vi "FPGA - PWM Example.vi"() -> ()   [LabVIEW 2013]
uses:
  <vilib>/rvi/Emulation/niFpgaSctlEmulationGetInTimedLoop.vi
  <vilib>/rvi/Emulation/niFpgaEmulationReportErrorSimple.vi
  <vilib>/rvi/Emulation/niFpgaProcessEmulError.vi
  <vilib>/rvi/Emulation/niFpgaGetClockAttributes.vi
  <vilib>/rvi/eio/common/nirviEmuTemplateMethod_errors.vi
  <vilib>/rvi/Emulation/niFpgaCriticalErrorInLSC.vi
  <vilib>/eio/EIONode/EIONode.xnode
panel:
  in  "PWM Duty Cycle (Ticks) 64":i32
  in  "PWM Duty Cycle (Ticks) 63":i32
  in  "PWM Duty Cycle (Ticks) 62":i32
  in  "PWM Duty Cycle (Ticks) 61":i32
  in  "PWM Duty Cycle (Ticks) 60":i32
  in  "PWM Duty Cycle (Ticks) 59":i32
  in  "PWM Duty Cycle (Ticks) 58":i32
  in  "PWM Duty Cycle (Ticks) 57":i32
  in  "PWM Duty Cycle (Ticks) 56":i32
  in  "PWM Duty Cycle (Ticks) 55":i32
  in  "PWM Duty Cycle (Ticks) 54":i32
  in  "PWM Duty Cycle (Ticks) 53":i32
  in  "PWM Duty Cycle (Ticks) 52":i32
  in  "PWM Duty Cycle (Ticks) 51":i32
  in  "PWM Duty Cycle (Ticks) 50":i32
  in  "PWM Duty Cycle (Ticks) 49":i32
  in  "PWM Duty Cycle (Ticks) 48":i32
  in  "PWM Duty Cycle (Ticks) 47":i32
  in  "PWM Duty Cycle (Ticks) 46":i32
  in  "PWM Duty Cycle (Ticks) 45":i32
  in  "PWM Duty Cycle (Ticks) 44":i32
  in  "PWM Duty Cycle (Ticks) 43":i32
  in  "PWM Duty Cycle (Ticks) 42":i32
  in  "PWM Duty Cycle (Ticks) 41":i32
  in  "PWM Duty Cycle (Ticks) 40":i32
  in  "PWM Duty Cycle (Ticks) 39":i32
  in  "PWM Duty Cycle (Ticks) 38":i32
  in  "PWM Duty Cycle (Ticks) 37":i32
  in  "PWM Duty Cycle (Ticks) 36":i32
  in  "PWM Duty Cycle (Ticks) 35":i32
  in  "PWM Duty Cycle (Ticks) 34":i32
  in  "PWM Duty Cycle (Ticks) 33":i32
  in  "PWM Duty Cycle (Ticks) 32":i32
  in  "PWM Duty Cycle (Ticks) 31":i32
  in  "PWM Duty Cycle (Ticks) 30":i32
  in  "PWM Duty Cycle (Ticks) 29":i32
  in  "PWM Duty Cycle (Ticks) 28":i32
  in  "PWM Duty Cycle (Ticks) 27":i32
  in  "PWM Duty Cycle (Ticks) 26":i32
  in  "PWM Duty Cycle (Ticks) 25":i32
  in  "PWM Duty Cycle (Ticks) 24":i32
  in  "PWM Duty Cycle (Ticks) 23":i32
  in  "PWM Duty Cycle (Ticks) 22":i32
  in  "PWM Duty Cycle (Ticks) 21":i32
  in  "PWM Duty Cycle (Ticks) 20":i32
  in  "PWM Duty Cycle (Ticks) 19":i32
  in  "PWM Duty Cycle (Ticks) 18":i32
  in  "PWM Duty Cycle (Ticks) 17":i32
  in  "PWM Duty Cycle (Ticks) 16":i32
  in  "PWM Duty Cycle (Ticks) 15":i32
  in  "PWM Duty Cycle (Ticks) 14":i32
  in  "PWM Duty Cycle (Ticks) 13":i32
  in  "PWM Duty Cycle (Ticks) 12":i32
  in  "PWM Duty Cycle (Ticks) 11":i32
  in  "PWM Duty Cycle (Ticks) 10":i32
  in  "PWM Duty Cycle (Ticks) 9":i32
  in  "PWM Duty Cycle (Ticks) 8":i32
  in  "PWM Duty Cycle (Ticks) 7":i32
  in  "PWM Duty Cycle (Ticks) 6":i32
  in  "PWM Duty Cycle (Ticks) 5":i32
  in  "PWM Duty Cycle (Ticks) 4":i32
  in  "PWM Duty Cycle (Ticks) 3":i32
  out "Rate (Ticks) 0..1":u32
  out "Telapsed (Ticks) 0..1":u32
  out "PWM Clock 0..1":bool
  out "9401/Slot 3 Error Code":i32
  out "stopped":bool
  in  "stop":bool
  in  "PWM Duty Cycle (Ticks) 2":i32
  in  "PWM Duty Cycle (Ticks) 1":i32
  in  "PWM Period (Ticks) 0..1":u32=40000
  # "NI 9401 PWM (Slot 3)"
  # "<- 1 Hz default"
  # "Error Codes\n65536 = Unable to communicate with module. \n65537 = Wrong module installed in slot."
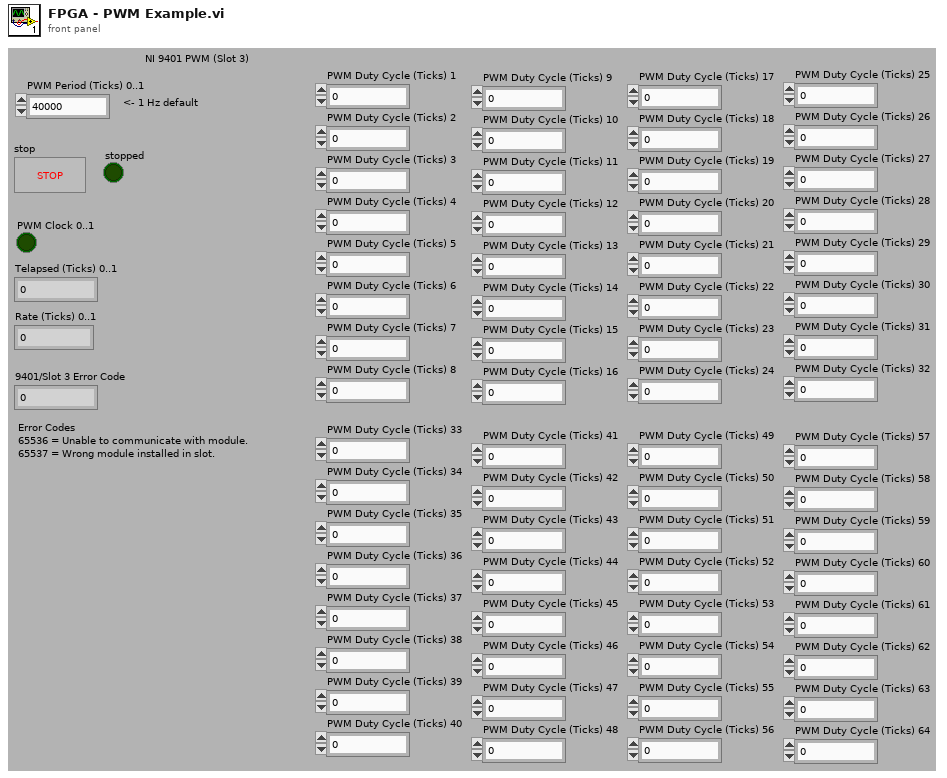
[diagram p1: front panel]
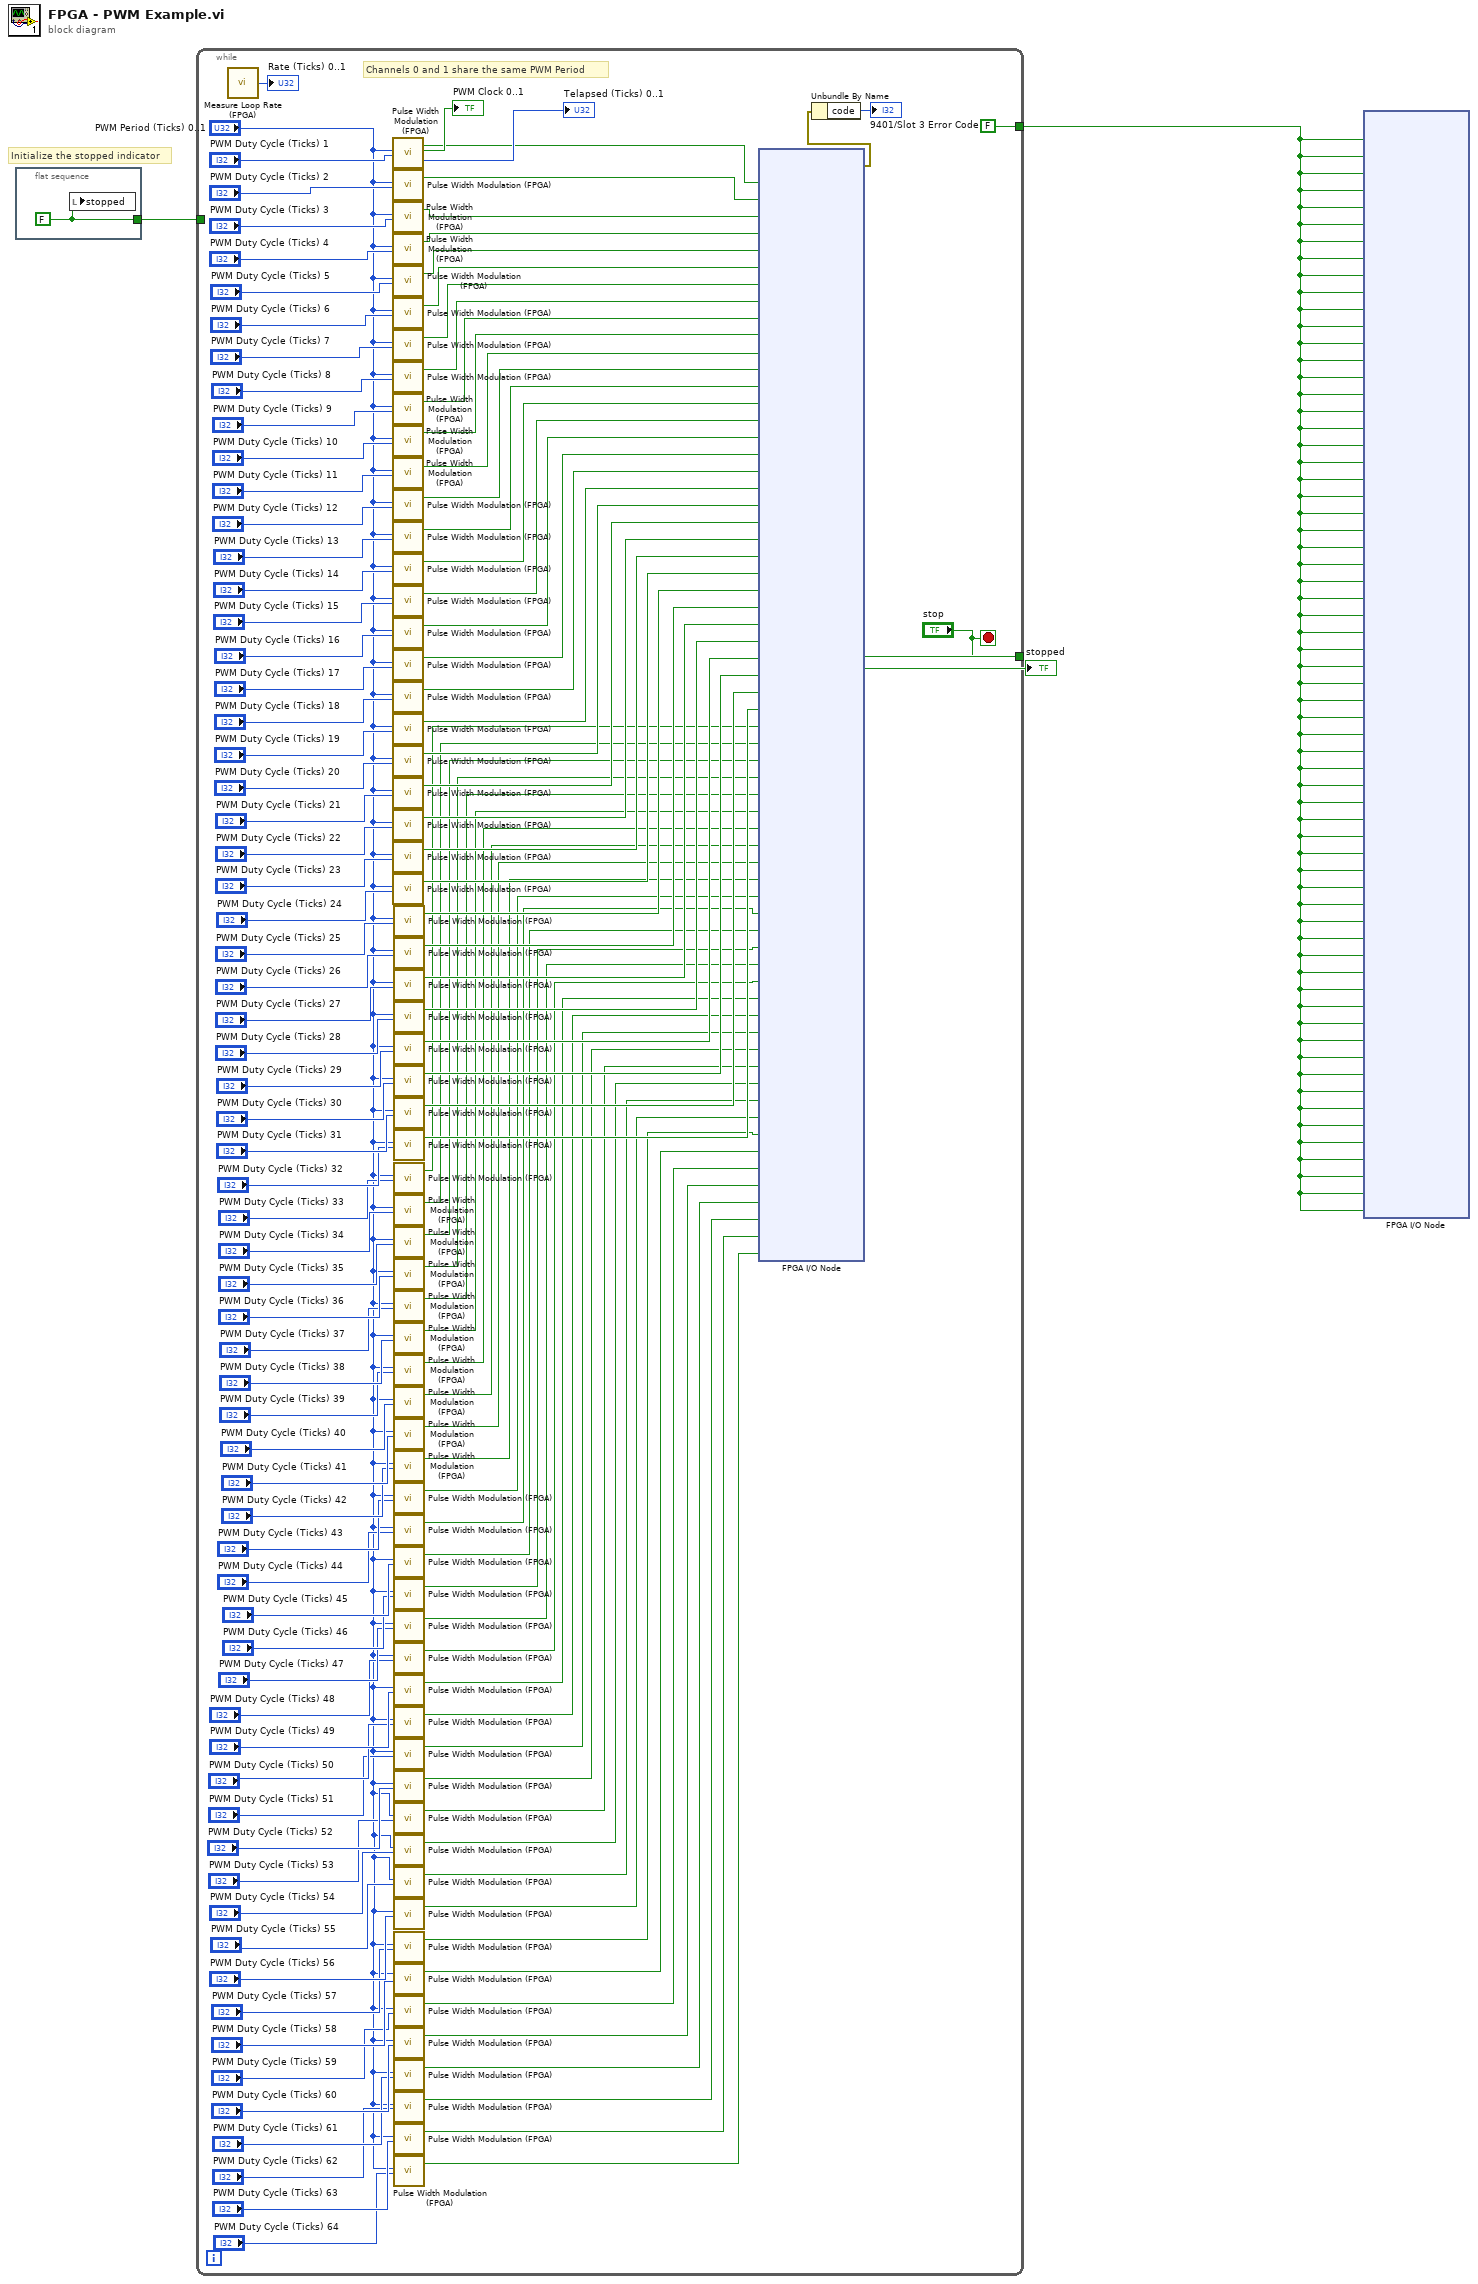
[diagram p0: block diagram]
diagram:
  # "Initialize the stopped indicator"
  n1 = flat-sequence {
    tunnel: [w4] -> w2
    frame #0 {
      w4 = FALSE ("stopped")
      n2 = local write "stopped"(w4) -> ()
    }
  }
  n3 = while {
    tunnel: [FALSE ("DO0")] -> w1
    tunnel: ["stop"] -> w3
    tunnel: w2 -> [_]
    stop <- "stop" stop-if-true
    # "Channels 0 and 1 share the same PWM Period"
    n4 = call "Measure Loop Rate (FPGA).vi"() -> ("Rate (Ticks)"=→"Rate (Ticks) 0..1":u32)  [unwired: 1 in]
    n5 = call "Pulse Width Modulation (FPGA).vi"("PWM Period (Ticks)"="PWM Period (Ticks) 0..1", "PWM Duty Cycle (Ticks)"="PWM Duty Cycle (Ticks) 1") -> ("PWM DO"=w125:bool, "PWM Clock"=→"PWM Clock 0..1":bool, "Telapsed (Ticks)"=→"Telapsed (Ticks) 0..1":u32)  [unwired: 14 in, 1 out]
    n6 = call "Pulse Width Modulation (FPGA).vi"("PWM Period (Ticks)"="PWM Period (Ticks) 0..1", "PWM Duty Cycle (Ticks)"="PWM Duty Cycle (Ticks) 2") -> ("PWM DO"=w124:bool)  [unwired: 14 in, 3 out]
    n7 = call "Pulse Width Modulation (FPGA).vi"("PWM Period (Ticks)"="PWM Period (Ticks) 0..1", "PWM Duty Cycle (Ticks)"="PWM Duty Cycle (Ticks) 3") -> ("PWM DO"=w123:bool)  [unwired: 14 in, 3 out]
    n8 = call "Pulse Width Modulation (FPGA).vi"("PWM Period (Ticks)"="PWM Period (Ticks) 0..1", "PWM Duty Cycle (Ticks)"="PWM Duty Cycle (Ticks) 4") -> ("PWM DO"=w122:bool)  [unwired: 14 in, 3 out]
    n9 = call "Pulse Width Modulation (FPGA).vi"("PWM Period (Ticks)"="PWM Period (Ticks) 0..1", "PWM Duty Cycle (Ticks)"="PWM Duty Cycle (Ticks) 5") -> ("PWM DO"=w121:bool)  [unwired: 14 in, 3 out]
    n10 = call "Pulse Width Modulation (FPGA).vi"("PWM Period (Ticks)"="PWM Period (Ticks) 0..1", "PWM Duty Cycle (Ticks)"="PWM Duty Cycle (Ticks) 6") -> ("PWM DO"=w120:bool)  [unwired: 14 in, 3 out]
    n11 = call "Pulse Width Modulation (FPGA).vi"("PWM Period (Ticks)"="PWM Period (Ticks) 0..1", "PWM Duty Cycle (Ticks)"="PWM Duty Cycle (Ticks) 7") -> ("PWM DO"=w119:bool)  [unwired: 14 in, 3 out]
    n12 = call "Pulse Width Modulation (FPGA).vi"("PWM Period (Ticks)"="PWM Period (Ticks) 0..1", "PWM Duty Cycle (Ticks)"="PWM Duty Cycle (Ticks) 8") -> ("PWM DO"=w118:bool)  [unwired: 14 in, 3 out]
    n13 = call "Pulse Width Modulation (FPGA).vi"("PWM Period (Ticks)"="PWM Period (Ticks) 0..1", "PWM Duty Cycle (Ticks)"="PWM Duty Cycle (Ticks) 9") -> ("PWM DO"=w117:bool)  [unwired: 14 in, 3 out]
    n14 = call "Pulse Width Modulation (FPGA).vi"("PWM Period (Ticks)"="PWM Period (Ticks) 0..1", "PWM Duty Cycle (Ticks)"="PWM Duty Cycle (Ticks) 10") -> ("PWM DO"=w116:bool)  [unwired: 14 in, 3 out]
    n15 = call "Pulse Width Modulation (FPGA).vi"("PWM Period (Ticks)"="PWM Period (Ticks) 0..1", "PWM Duty Cycle (Ticks)"="PWM Duty Cycle (Ticks) 11") -> ("PWM DO"=w115:bool)  [unwired: 14 in, 3 out]
    n16 = call "Pulse Width Modulation (FPGA).vi"("PWM Period (Ticks)"="PWM Period (Ticks) 0..1", "PWM Duty Cycle (Ticks)"="PWM Duty Cycle (Ticks) 12") -> ("PWM DO"=w114:bool)  [unwired: 14 in, 3 out]
    n17 = call "Pulse Width Modulation (FPGA).vi"("PWM Period (Ticks)"="PWM Period (Ticks) 0..1", "PWM Duty Cycle (Ticks)"="PWM Duty Cycle (Ticks) 13") -> ("PWM DO"=w113:bool)  [unwired: 14 in, 3 out]
    n18 = call "Pulse Width Modulation (FPGA).vi"("PWM Period (Ticks)"="PWM Period (Ticks) 0..1", "PWM Duty Cycle (Ticks)"="PWM Duty Cycle (Ticks) 14") -> ("PWM DO"=w112:bool)  [unwired: 14 in, 3 out]
    n19 = call "Pulse Width Modulation (FPGA).vi"("PWM Period (Ticks)"="PWM Period (Ticks) 0..1", "PWM Duty Cycle (Ticks)"="PWM Duty Cycle (Ticks) 15") -> ("PWM DO"=w111:bool)  [unwired: 14 in, 3 out]
    n20 = call "Pulse Width Modulation (FPGA).vi"("PWM Period (Ticks)"="PWM Period (Ticks) 0..1", "PWM Duty Cycle (Ticks)"="PWM Duty Cycle (Ticks) 16") -> ("PWM DO"=w110:bool)  [unwired: 14 in, 3 out]
    n21 = call "Pulse Width Modulation (FPGA).vi"("PWM Period (Ticks)"="PWM Period (Ticks) 0..1", "PWM Duty Cycle (Ticks)"="PWM Duty Cycle (Ticks) 17") -> ("PWM DO"=w109:bool)  [unwired: 14 in, 3 out]
    n22 = call "Pulse Width Modulation (FPGA).vi"("PWM Period (Ticks)"="PWM Period (Ticks) 0..1", "PWM Duty Cycle (Ticks)"="PWM Duty Cycle (Ticks) 18") -> ("PWM DO"=w108:bool)  [unwired: 14 in, 3 out]
    n23 = call "Pulse Width Modulation (FPGA).vi"("PWM Period (Ticks)"="PWM Period (Ticks) 0..1", "PWM Duty Cycle (Ticks)"="PWM Duty Cycle (Ticks) 19") -> ("PWM DO"=w107:bool)  [unwired: 14 in, 3 out]
    n24 = call "Pulse Width Modulation (FPGA).vi"("PWM Period (Ticks)"="PWM Period (Ticks) 0..1", "PWM Duty Cycle (Ticks)"="PWM Duty Cycle (Ticks) 20") -> ("PWM DO"=w106:bool)  [unwired: 14 in, 3 out]
    n25 = call "Pulse Width Modulation (FPGA).vi"("PWM Period (Ticks)"="PWM Period (Ticks) 0..1", "PWM Duty Cycle (Ticks)"="PWM Duty Cycle (Ticks) 21") -> ("PWM DO"=w105:bool)  [unwired: 14 in, 3 out]
    n26 = call "Pulse Width Modulation (FPGA).vi"("PWM Period (Ticks)"="PWM Period (Ticks) 0..1", "PWM Duty Cycle (Ticks)"="PWM Duty Cycle (Ticks) 22") -> ("PWM DO"=w104:bool)  [unwired: 14 in, 3 out]
    n27 = call "Pulse Width Modulation (FPGA).vi"("PWM Period (Ticks)"="PWM Period (Ticks) 0..1", "PWM Duty Cycle (Ticks)"="PWM Duty Cycle (Ticks) 23") -> ("PWM DO"=w103:bool)  [unwired: 14 in, 3 out]
    n28 = call "Pulse Width Modulation (FPGA).vi"("PWM Period (Ticks)"="PWM Period (Ticks) 0..1", "PWM Duty Cycle (Ticks)"="PWM Duty Cycle (Ticks) 24") -> ("PWM DO"=w102:bool)  [unwired: 14 in, 3 out]
    n29 = call "Pulse Width Modulation (FPGA).vi"("PWM Period (Ticks)"="PWM Period (Ticks) 0..1", "PWM Duty Cycle (Ticks)"="PWM Duty Cycle (Ticks) 25") -> ("PWM DO"=w101:bool)  [unwired: 14 in, 3 out]
    n30 = call "Pulse Width Modulation (FPGA).vi"("PWM Period (Ticks)"="PWM Period (Ticks) 0..1", "PWM Duty Cycle (Ticks)"="PWM Duty Cycle (Ticks) 26") -> ("PWM DO"=w100:bool)  [unwired: 14 in, 3 out]
    n31 = call "Pulse Width Modulation (FPGA).vi"("PWM Period (Ticks)"="PWM Period (Ticks) 0..1", "PWM Duty Cycle (Ticks)"="PWM Duty Cycle (Ticks) 27") -> ("PWM DO"=w99:bool)  [unwired: 14 in, 3 out]
    n32 = call "Pulse Width Modulation (FPGA).vi"("PWM Period (Ticks)"="PWM Period (Ticks) 0..1", "PWM Duty Cycle (Ticks)"="PWM Duty Cycle (Ticks) 28") -> ("PWM DO"=w98:bool)  [unwired: 14 in, 3 out]
    n33 = call "Pulse Width Modulation (FPGA).vi"("PWM Period (Ticks)"="PWM Period (Ticks) 0..1", "PWM Duty Cycle (Ticks)"="PWM Duty Cycle (Ticks) 29") -> ("PWM DO"=w97:bool)  [unwired: 14 in, 3 out]
    n34 = call "Pulse Width Modulation (FPGA).vi"("PWM Period (Ticks)"="PWM Period (Ticks) 0..1", "PWM Duty Cycle (Ticks)"="PWM Duty Cycle (Ticks) 30") -> ("PWM DO"=w96:bool)  [unwired: 14 in, 3 out]
    n35 = call "Pulse Width Modulation (FPGA).vi"("PWM Period (Ticks)"="PWM Period (Ticks) 0..1", "PWM Duty Cycle (Ticks)"="PWM Duty Cycle (Ticks) 31") -> ("PWM DO"=w95:bool)  [unwired: 14 in, 3 out]
    n36 = call "Pulse Width Modulation (FPGA).vi"("PWM Period (Ticks)"="PWM Period (Ticks) 0..1", "PWM Duty Cycle (Ticks)"="PWM Duty Cycle (Ticks) 32") -> ("PWM DO"=w94:bool)  [unwired: 14 in, 3 out]
    n37 = call "Pulse Width Modulation (FPGA).vi"("PWM Period (Ticks)"="PWM Period (Ticks) 0..1", "PWM Duty Cycle (Ticks)"="PWM Duty Cycle (Ticks) 33") -> ("PWM DO"=w93:bool)  [unwired: 14 in, 3 out]
    n38 = call "Pulse Width Modulation (FPGA).vi"("PWM Period (Ticks)"="PWM Period (Ticks) 0..1", "PWM Duty Cycle (Ticks)"="PWM Duty Cycle (Ticks) 34") -> ("PWM DO"=w92:bool)  [unwired: 14 in, 3 out]
    n39 = call "Pulse Width Modulation (FPGA).vi"("PWM Period (Ticks)"="PWM Period (Ticks) 0..1", "PWM Duty Cycle (Ticks)"="PWM Duty Cycle (Ticks) 35") -> ("PWM DO"=w91:bool)  [unwired: 14 in, 3 out]
    n40 = call "Pulse Width Modulation (FPGA).vi"("PWM Period (Ticks)"="PWM Period (Ticks) 0..1", "PWM Duty Cycle (Ticks)"="PWM Duty Cycle (Ticks) 36") -> ("PWM DO"=w90:bool)  [unwired: 14 in, 3 out]
    n41 = call "Pulse Width Modulation (FPGA).vi"("PWM Period (Ticks)"="PWM Period (Ticks) 0..1", "PWM Duty Cycle (Ticks)"="PWM Duty Cycle (Ticks) 37") -> ("PWM DO"=w89:bool)  [unwired: 14 in, 3 out]
    n42 = call "Pulse Width Modulation (FPGA).vi"("PWM Period (Ticks)"="PWM Period (Ticks) 0..1", "PWM Duty Cycle (Ticks)"="PWM Duty Cycle (Ticks) 38") -> ("PWM DO"=w88:bool)  [unwired: 14 in, 3 out]
    n43 = call "Pulse Width Modulation (FPGA).vi"("PWM Period (Ticks)"="PWM Period (Ticks) 0..1", "PWM Duty Cycle (Ticks)"="PWM Duty Cycle (Ticks) 39") -> ("PWM DO"=w87:bool)  [unwired: 14 in, 3 out]
    n44 = call "Pulse Width Modulation (FPGA).vi"("PWM Period (Ticks)"="PWM Period (Ticks) 0..1", "PWM Duty Cycle (Ticks)"="PWM Duty Cycle (Ticks) 40") -> ("PWM DO"=w86:bool)  [unwired: 14 in, 3 out]
    n45 = call "Pulse Width Modulation (FPGA).vi"("PWM Period (Ticks)"="PWM Period (Ticks) 0..1", "PWM Duty Cycle (Ticks)"="PWM Duty Cycle (Ticks) 41") -> ("PWM DO"=w85:bool)  [unwired: 14 in, 3 out]
    n46 = call "Pulse Width Modulation (FPGA).vi"("PWM Period (Ticks)"="PWM Period (Ticks) 0..1", "PWM Duty Cycle (Ticks)"="PWM Duty Cycle (Ticks) 42") -> ("PWM DO"=w84:bool)  [unwired: 14 in, 3 out]
    n47 = call "Pulse Width Modulation (FPGA).vi"("PWM Period (Ticks)"="PWM Period (Ticks) 0..1", "PWM Duty Cycle (Ticks)"="PWM Duty Cycle (Ticks) 43") -> ("PWM DO"=w83:bool)  [unwired: 14 in, 3 out]
    n48 = call "Pulse Width Modulation (FPGA).vi"("PWM Period (Ticks)"="PWM Period (Ticks) 0..1", "PWM Duty Cycle (Ticks)"="PWM Duty Cycle (Ticks) 44") -> ("PWM DO"=w82:bool)  [unwired: 14 in, 3 out]
    n49 = call "Pulse Width Modulation (FPGA).vi"("PWM Period (Ticks)"="PWM Period (Ticks) 0..1", "PWM Duty Cycle (Ticks)"="PWM Duty Cycle (Ticks) 45") -> ("PWM DO"=w81:bool)  [unwired: 14 in, 3 out]
    n50 = call "Pulse Width Modulation (FPGA).vi"("PWM Period (Ticks)"="PWM Period (Ticks) 0..1", "PWM Duty Cycle (Ticks)"="PWM Duty Cycle (Ticks) 46") -> ("PWM DO"=w80:bool)  [unwired: 14 in, 3 out]
    n51 = call "Pulse Width Modulation (FPGA).vi"("PWM Period (Ticks)"="PWM Period (Ticks) 0..1", "PWM Duty Cycle (Ticks)"="PWM Duty Cycle (Ticks) 47") -> ("PWM DO"=w79:bool)  [unwired: 14 in, 3 out]
    n52 = call "Pulse Width Modulation (FPGA).vi"("PWM Period (Ticks)"="PWM Period (Ticks) 0..1", "PWM Duty Cycle (Ticks)"="PWM Duty Cycle (Ticks) 48") -> ("PWM DO"=w78:bool)  [unwired: 14 in, 3 out]
    n53 = call "Pulse Width Modulation (FPGA).vi"("PWM Period (Ticks)"="PWM Period (Ticks) 0..1", "PWM Duty Cycle (Ticks)"="PWM Duty Cycle (Ticks) 49") -> ("PWM DO"=w77:bool)  [unwired: 14 in, 3 out]
    n54 = call "Pulse Width Modulation (FPGA).vi"("PWM Period (Ticks)"="PWM Period (Ticks) 0..1", "PWM Duty Cycle (Ticks)"="PWM Duty Cycle (Ticks) 50") -> ("PWM DO"=w76:bool)  [unwired: 14 in, 3 out]
    n55 = call "Pulse Width Modulation (FPGA).vi"("PWM Period (Ticks)"="PWM Period (Ticks) 0..1", "PWM Duty Cycle (Ticks)"="PWM Duty Cycle (Ticks) 51") -> ("PWM DO"=w75:bool)  [unwired: 14 in, 3 out]
    n56 = call "Pulse Width Modulation (FPGA).vi"("PWM Period (Ticks)"="PWM Period (Ticks) 0..1", "PWM Duty Cycle (Ticks)"="PWM Duty Cycle (Ticks) 52") -> ("PWM DO"=w74:bool)  [unwired: 14 in, 3 out]
    n57 = call "Pulse Width Modulation (FPGA).vi"("PWM Period (Ticks)"="PWM Period (Ticks) 0..1", "PWM Duty Cycle (Ticks)"="PWM Duty Cycle (Ticks) 53") -> ("PWM DO"=w73:bool)  [unwired: 14 in, 3 out]
    n58 = call "Pulse Width Modulation (FPGA).vi"("PWM Period (Ticks)"="PWM Period (Ticks) 0..1", "PWM Duty Cycle (Ticks)"="PWM Duty Cycle (Ticks) 54") -> ("PWM DO"=w72:bool)  [unwired: 14 in, 3 out]
    n59 = call "Pulse Width Modulation (FPGA).vi"("PWM Period (Ticks)"="PWM Period (Ticks) 0..1", "PWM Duty Cycle (Ticks)"="PWM Duty Cycle (Ticks) 55") -> ("PWM DO"=w71:bool)  [unwired: 14 in, 3 out]
    n60 = call "Pulse Width Modulation (FPGA).vi"("PWM Period (Ticks)"="PWM Period (Ticks) 0..1", "PWM Duty Cycle (Ticks)"="PWM Duty Cycle (Ticks) 56") -> ("PWM DO"=w70:bool)  [unwired: 14 in, 3 out]
    n61 = call "Pulse Width Modulation (FPGA).vi"("PWM Period (Ticks)"="PWM Period (Ticks) 0..1", "PWM Duty Cycle (Ticks)"="PWM Duty Cycle (Ticks) 57") -> ("PWM DO"=w69:bool)  [unwired: 14 in, 3 out]
    n62 = call "Pulse Width Modulation (FPGA).vi"("PWM Period (Ticks)"="PWM Period (Ticks) 0..1", "PWM Duty Cycle (Ticks)"="PWM Duty Cycle (Ticks) 58") -> ("PWM DO"=w68:bool)  [unwired: 14 in, 3 out]
    n63 = call "Pulse Width Modulation (FPGA).vi"("PWM Period (Ticks)"="PWM Period (Ticks) 0..1", "PWM Duty Cycle (Ticks)"="PWM Duty Cycle (Ticks) 59") -> ("PWM DO"=w67:bool)  [unwired: 14 in, 3 out]
    n64 = call "Pulse Width Modulation (FPGA).vi"("PWM Period (Ticks)"="PWM Period (Ticks) 0..1", "PWM Duty Cycle (Ticks)"="PWM Duty Cycle (Ticks) 60") -> ("PWM DO"=w66:bool)  [unwired: 14 in, 3 out]
    n65 = call "Pulse Width Modulation (FPGA).vi"("PWM Period (Ticks)"="PWM Period (Ticks) 0..1", "PWM Duty Cycle (Ticks)"="PWM Duty Cycle (Ticks) 61") -> ("PWM DO"=w65:bool)  [unwired: 14 in, 3 out]
    n66 = call "Pulse Width Modulation (FPGA).vi"("PWM Period (Ticks)"="PWM Period (Ticks) 0..1", "PWM Duty Cycle (Ticks)"="PWM Duty Cycle (Ticks) 62") -> ("PWM DO"=w64:bool)  [unwired: 14 in, 3 out]
    n67 = call "Pulse Width Modulation (FPGA).vi"("PWM Period (Ticks)"="PWM Period (Ticks) 0..1", "PWM Duty Cycle (Ticks)"="PWM Duty Cycle (Ticks) 63") -> ("PWM DO"=w63:bool)  [unwired: 14 in, 3 out]
    n68 = call "Pulse Width Modulation (FPGA).vi"("PWM Period (Ticks)"="PWM Period (Ticks) 0..1", "PWM Duty Cycle (Ticks)"="PWM Duty Cycle (Ticks) 64") -> ("PWM DO"=w62:bool)  [unwired: 14 in, 3 out]
    n69 = xnode "FPGA I/O Node"("Mod1/DIO0"=w125, "Mod1/DIO1"=w124, "Mod1/DIO2"=w123, "Mod1/DIO3"=w122, "Mod1/DIO4"=w121, "Mod1/DIO5"=w120, "Mod1/DIO6"=w119, "Mod1/DIO7"=w118, "Mod2/DIO0"=w117, "Mod2/DIO1"=w116, "Mod2/DIO2"=w115, "Mod2/DIO3"=w114, "Mod2/DIO4"=w113, "Mod2/DIO5"=w112, "Mod2/DIO6"=w111, "Mod2/DIO7"=w110, "Mod3/DIO0"=w109, "Mod3/DIO1"=w108, "Mod3/DIO2"=w107, "Mod3/DIO3"=w106, "Mod3/DIO4"=w105, "Mod3/DIO5"=w104, "Mod3/DIO6"=w103, "Mod3/DIO7"=w102, "Mod4/DIO0"=w101, "Mod4/DIO1"=w100, "Mod4/DIO2"=w99, "Mod4/DIO3"=w98, "Mod4/DIO4"=w97, "Mod4/DIO5"=w96, "Mod4/DIO6"=w95, "Mod4/DIO7"=w94, "Mod5/DIO0"=w93, "Mod5/DIO1"=w92, "Mod5/DIO2"=w91, "Mod5/DIO3"=w90, "Mod5/DIO4"=w89, "Mod5/DIO5"=w88, "Mod5/DIO6"=w87, "Mod5/DIO7"=w86, "Mod6/DIO0"=w85, "Mod6/DIO1"=w84, "Mod6/DIO2"=w83, "Mod6/DIO3"=w82, "Mod6/DIO4"=w81, "Mod6/DIO5"=w80, "Mod6/DIO6"=w79, "Mod6/DIO7"=w78, "Mod7/DIO0"=w77, "Mod7/DIO1"=w76, "Mod7/DIO2"=w75, "Mod7/DIO3"=w74, "Mod7/DIO4"=w73, "Mod7/DIO5"=w72, "Mod7/DIO6"=w71, "Mod7/DIO7"=w70, "Mod8/DIO0"=w69, "Mod8/DIO1"=w68, "Mod8/DIO2"=w67, "Mod8/DIO3"=w66, "Mod8/DIO4"=w65, "Mod8/DIO5"=w64, "Mod8/DIO6"=w63, "Mod8/DIO7"=w62) -> ("error out"=w136:errorcluster)  [unwired: 65 in, 64 out]
    n70 = Unbundle By Name(w136) -> ("code"=→"9401/Slot 3 Error Code":i32)
  }
  "stopped" <- w3
  n71 = xnode "FPGA I/O Node"("Mod1/DIO0"=w1, "Mod1/DIO1"=w1, "Mod1/DIO2"=w1, "Mod1/DIO3"=w1, "Mod1/DIO4"=w1, "Mod1/DIO5"=w1, "Mod1/DIO6"=w1, "Mod1/DIO7"=w1, "Mod2/DIO0"=w1, "Mod2/DIO1"=w1, "Mod2/DIO2"=w1, "Mod2/DIO3"=w1, "Mod2/DIO4"=w1, "Mod2/DIO5"=w1, "Mod2/DIO6"=w1, "Mod2/DIO7"=w1, "Mod3/DIO0"=w1, "Mod3/DIO1"=w1, "Mod3/DIO2"=w1, "Mod3/DIO3"=w1, "Mod3/DIO4"=w1, "Mod3/DIO5"=w1, "Mod3/DIO6"=w1, "Mod3/DIO7"=w1, "Mod4/DIO0"=w1, "Mod4/DIO1"=w1, "Mod4/DIO2"=w1, "Mod4/DIO3"=w1, "Mod4/DIO4"=w1, "Mod4/DIO5"=w1, "Mod4/DIO6"=w1, "Mod4/DIO7"=w1, "Mod5/DIO0"=w1, "Mod5/DIO1"=w1, "Mod5/DIO2"=w1, "Mod5/DIO3"=w1, "Mod5/DIO4"=w1, "Mod5/DIO5"=w1, "Mod5/DIO6"=w1, "Mod5/DIO7"=w1, "Mod6/DIO0"=w1, "Mod6/DIO1"=w1, "Mod6/DIO2"=w1, "Mod6/DIO3"=w1, "Mod6/DIO4"=w1, "Mod6/DIO5"=w1, "Mod6/DIO6"=w1, "Mod6/DIO7"=w1, "Mod7/DIO0"=w1, "Mod7/DIO1"=w1, "Mod7/DIO2"=w1, "Mod7/DIO3"=w1, "Mod7/DIO4"=w1, "Mod7/DIO5"=w1, "Mod7/DIO6"=w1, "Mod7/DIO7"=w1, "Mod8/DIO0"=w1, "Mod8/DIO1"=w1, "Mod8/DIO2"=w1, "Mod8/DIO3"=w1, "Mod8/DIO4"=w1, "Mod8/DIO5"=w1, "Mod8/DIO6"=w1, "Mod8/DIO7"=w1) -> ()  [unwired: 64 in, 64 out]
